vi "CS SQL Client.Global.vi"(2 "Address":string="localhost", 3 "command":T1(ring)=enum."default") -> (0 "connection out":refnum<k5>)   [LabVIEW 2015, in "CS SQL Server.lvlib"]
doc: "This FGV VI is used to maintain the TCP/IP connection to the CS SQL Server.\n\nErrors are handled by \"CS SQL Client.vi\"."
uses:
  CS SQL Server.lvlib
  CSlibraries/UtilityLib/UtilityLib.lvlib
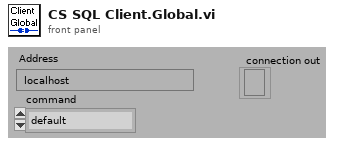
[diagram p1: front panel]
types:
  T1 = enum16{"connect", "disconnect", "reconnect", "default"}
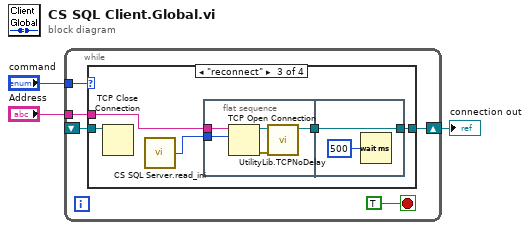
[diagram p0: block diagram]
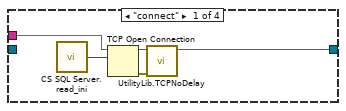
[diagram p2: hidden frame]
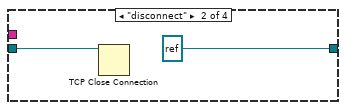
[diagram p3: hidden frame]
diagram:
  n1 = while {
    shift-right: [w8] -> w2
    shift-left: _ -> [w7]
    tunnel: "command" -> [w5]
    tunnel: "Address" -> [w4]
    stop <- TRUE stop-if-true
    n2 = case shown="\"reconnect\"" w5 {
      tunnel: w7 -> [_ w15 w20 w28]
      tunnel: [w11 refnum<k5> refnum ("connection out") w19 w28] -> w8
      tunnel: w4 -> [w10 _ w18 _]
      frame "connect" {
        n3 = call "CS SQL Server.read_ini.vi"() -> ("Port"=w9:u32)
        n4 = TCP Open Connection(address=w10, remote port or service name=w9) -> (connection ID=w13:refnum<k5>, error out=w12:errorcluster)  [unwired: 3 in]
        n5 = call "UtilityLib.TCPNoDelay.vi"("error in (no error)"=w12, "connection in"=w13) -> ("connection out"=w11:refnum<k5>)  [unwired: 8 in, 1 out]
      }
      frame "disconnect" {
        n6 = TCP Close Connection(connection ID=w15) -> ()  [unwired: 2 in, 2 out]
      }
      frame "reconnect" {
        n7 = TCP Close Connection(connection ID=w20) -> ()  [unwired: 2 in, 2 out]
        n8 = call "CS SQL Server.read_ini.vi"() -> ("Port"=w17:u32)
        n9 = flat-sequence {
          tunnel: [w24] -> w16
          tunnel: w18 -> [w23]
          tunnel: w17 -> [w22]
          tunnel: [w26] -> w19
          tunnel: w16 -> [w26]
          frame #0 {
            n10 = TCP Open Connection(address=w23, remote port or service name=w22) -> (connection ID=w25:refnum<k5>, error out=w21:errorcluster)  [unwired: 3 in]
            n11 = call "UtilityLib.TCPNoDelay.vi"("error in (no error)"=w21, "connection in"=w25) -> ("connection out"=w24:refnum<k5>)  [unwired: 8 in, 1 out]
          }
          frame #1 {
            n12 = Wait (ms)(milliseconds to wait=u32 500) -> ()  [unwired: 1 out]
          }
        }
      }
      frame Default {
      }
    }
  }
  "connection out" <- w2
